vi "Close Object.vi"(8 "error in (no error)":errorcluster, 11 "Switching Object":refnum<class "FPT_SParam_Switching.lvclass">) -> (0 "error out":errorcluster)   [LabVIEW 2023, in "FPT_SParam_Switching.lvclass"]
uses:
  FPT_SParam_Switching.lvclass
  FPT_SParam_Switching.lvclass/FPT_SParam_Switching.ctl
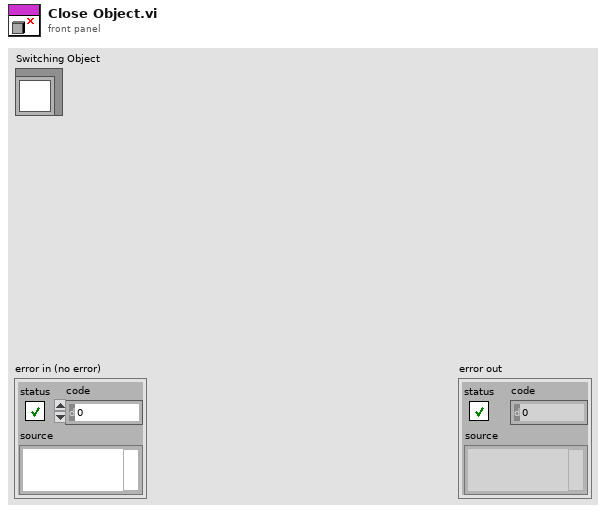
[diagram p1: front panel]
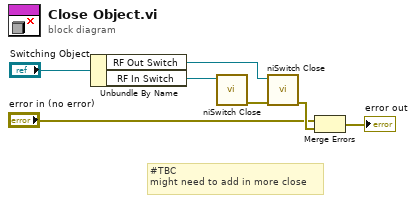
[diagram p0: block diagram]
diagram:
  # "#TBC\nmight need to add in more close"
  n1 = Unbundle By Name("Switching Object") -> ("RF Out Switch"=w5:refnum<k15>, "RF In Switch"=w6:refnum<k15>)
  n2 = call <instrlib>:"niSwitch Close.vi"("instrument handle"=w6) -> ("error out"=w4:errorcluster)  [unwired: 10 in]
  n3 = call <instrlib>:"niSwitch Close.vi"("error in (no error)"=w4, "instrument handle"=w5) -> ("error out"=w3:errorcluster)  [unwired: 9 in]
  n4 = Merge Errors("error in (no error)", w3) -> (→"error out":errorcluster)
